vi "Set Basic Config.vi"(10 "Module Data":string[][](array[string]), 11 "Config Data":string[][](array[string])) -> (3 "Config Out":string[][](array[string]))   [LabVIEW 2018]
panel:
  out "Array":string[][](array[string])
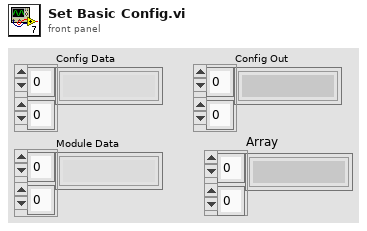
[diagram p1: front panel]
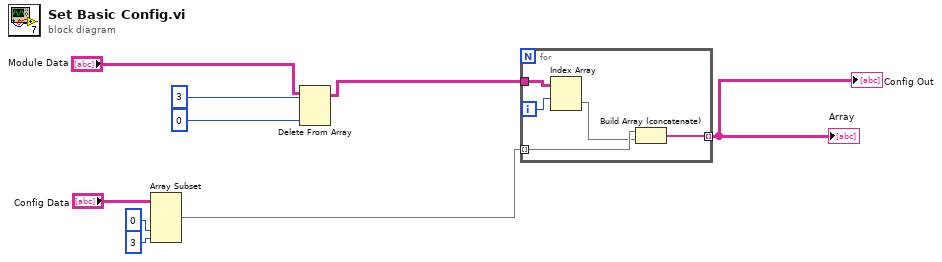
[diagram p0: block diagram]
diagram:
  n1 = Array Subset(array="Config Data", index (col)=0 ("index"), length (col)=3 ("length")) -> (w9:string[][])  [unwired: 2 in]
  n2 = Delete From Array(array="Module Data", length=3, index (col)=0 ("disabled index (col)")) -> (array with subset deleted=w2:string[][])  [unwired: 1 in, 1 out]
  n3 = for {
    tunnel: w9 -> [w12] mode=indexing
    tunnel: [w10] -> w1 mode=indexing
    tunnel: w2 -> [w13]
    i -> [w14]
    n4 = Index Array(array=w13, index (row)=w14) -> (element=w11:string[])  [unwired: 1 in]
    n5 = Build Array (concatenate)(w12, w11) -> (w10:string[])
  }
  "Config Out" <- w1
  "Array" <- w1
